vi "MiniWheel Simple Control Code Revised.vi"() -> ()   [LabVIEW 2016]
uses:
  <userlib>/dynamixel/dynamixel.lvlib
panel:
  in  "Baud Rate":i32=1
  in  "Com Port":i32=3
  in  "Goal Omega 2":u16=512 max=1023 step=1
  in  "Goal position 3":u16=512 max=1023 step=1
  in  "Wheel Dynamixel ID":i32=1
  out "Motor Position V. Time":i32(graph)
  in  "Rotator Dynamixel ID":i32=1
  in  "stop":bool
  out "Present Position":u16(slide) max=1023 scale=0.0..1023.0
  # "Instructions:\n1) Enter Initialization Parameters\n2) Enter Goal Omega and Goal Position\n3) Click \"START Motors\" button\n4) Change parameter values as desired during operation"
  # "Motor Feedback"
  # "Initialization"
  # "Parameters"
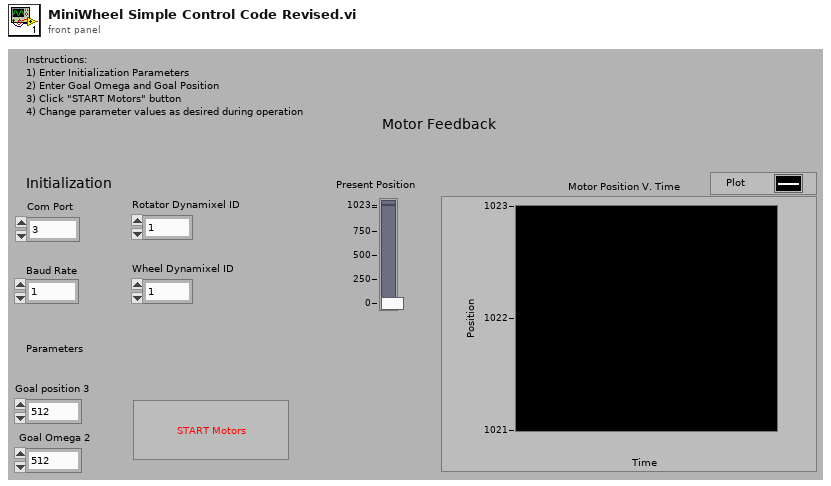
[diagram p1: front panel]
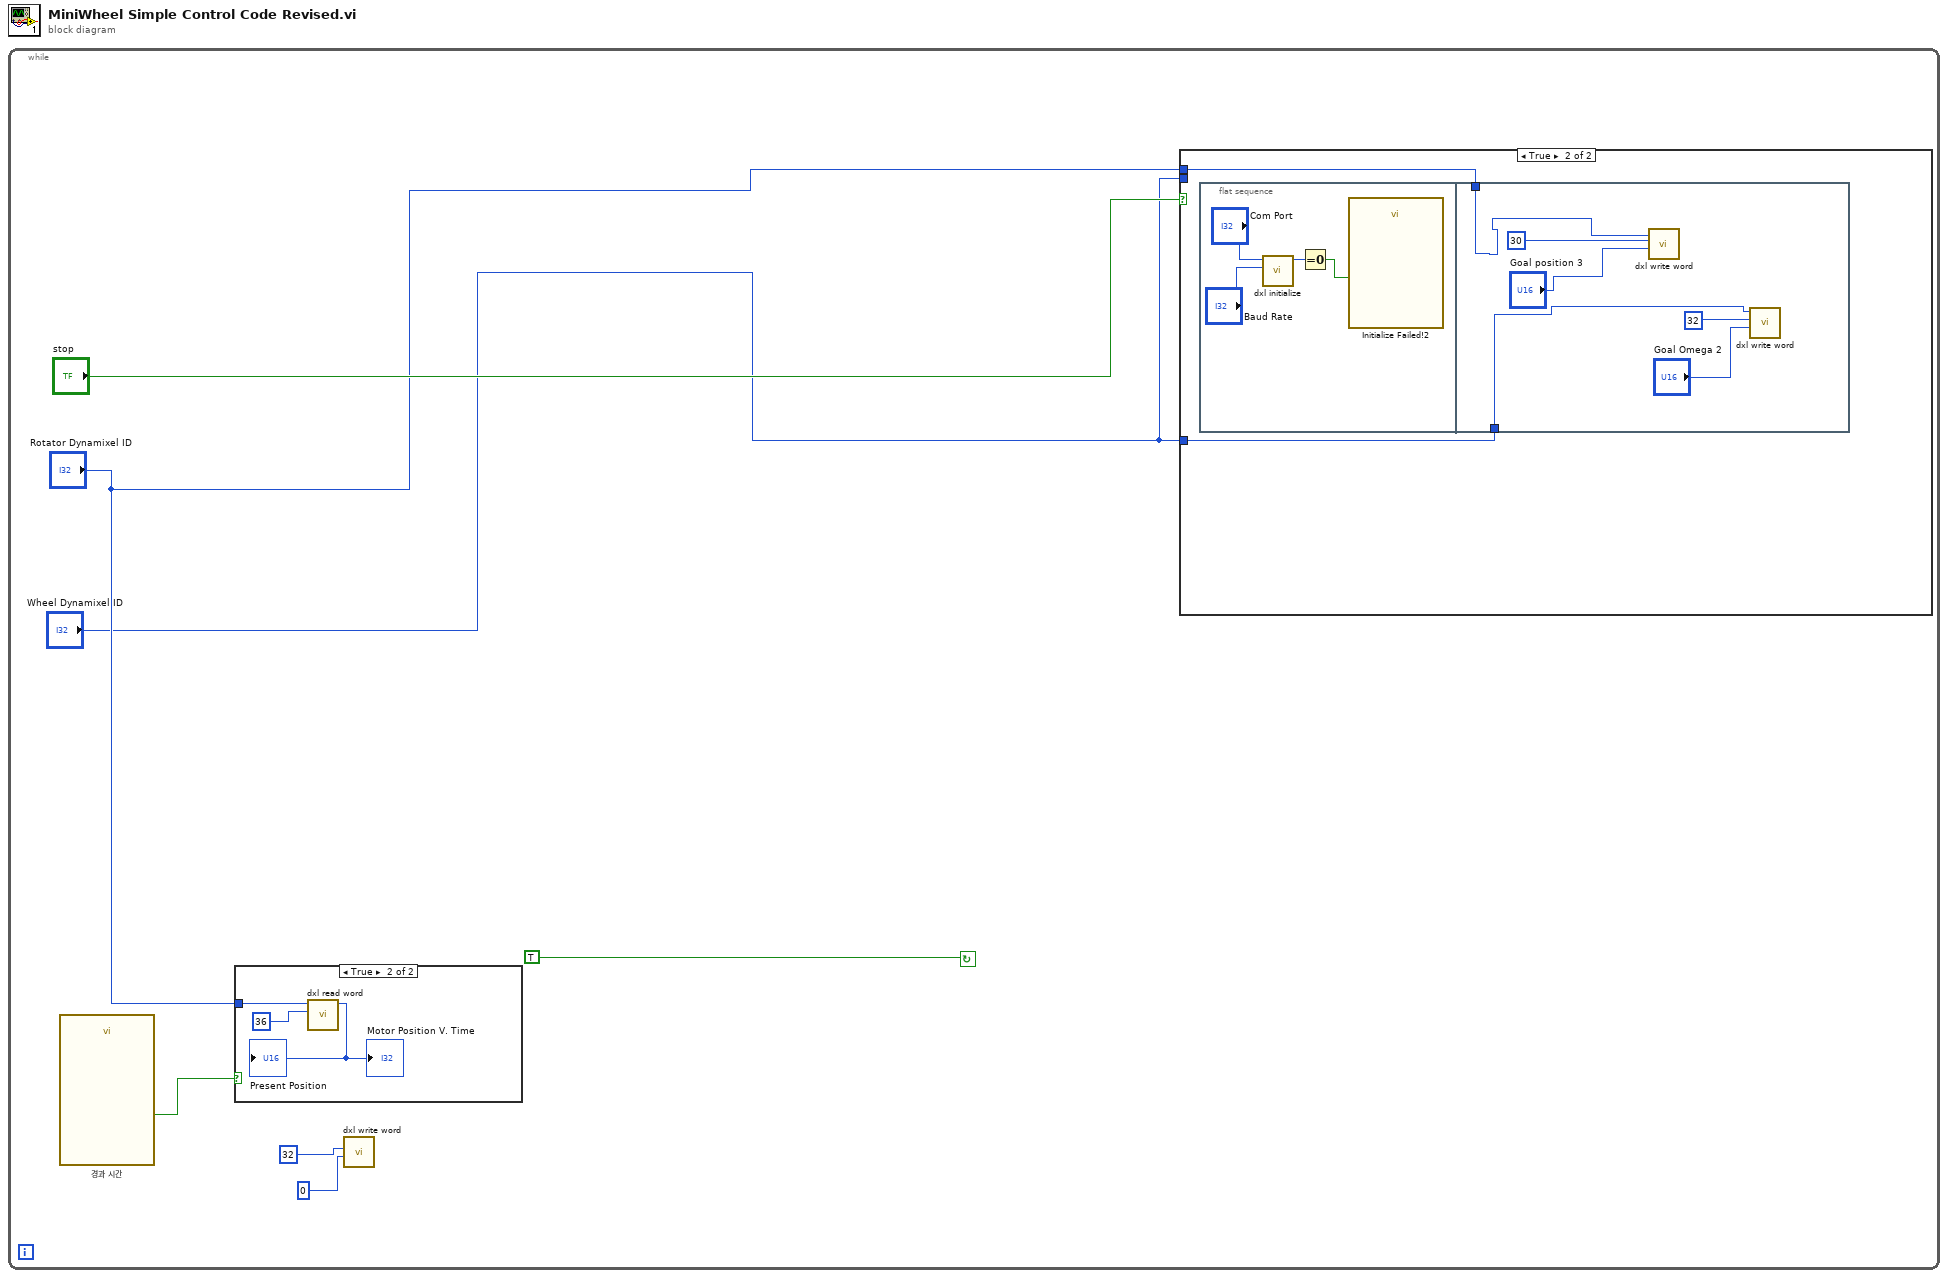
[diagram p0: block diagram]
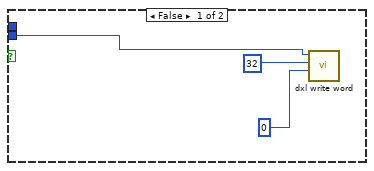
[diagram p2: hidden frame]
diagram:
  n1 = while {
    stop <- TRUE continue-if-true
    n2 = call "경과 시간"() -> ("Time has Elapsed"=w6:bool)  [unwired: 12 in, 7 out]
    n3 = case shown="True" w6 {
      tunnel: "Rotator Dynamixel ID" -> [_ w25]
      frame False {
      }
      frame True {
        n4 = call <userlib>:"dxl read word.vi"("address"=36, "id"=w25) -> ("function return"=→"Present Position" →"Motor Position V. Time":i32)  [unwired: 9 in]
      }
    }
    n5 = call <userlib>:"dxl write word.vi"("value"=0, "address"=32) -> ()  [unwired: 10 in]
    n6 = case shown="True" "stop" {
      tunnel: "Wheel Dynamixel ID" -> [w9 _]
      tunnel: "Rotator Dynamixel ID" -> [_ w12]
      tunnel: "Wheel Dynamixel ID" -> [_ w11]
      frame False {
        n7 = call <userlib>:"dxl write word.vi"("value"=0, "address"=32, "id"=w9) -> ()  [unwired: 9 in]
      }
      frame True {
        n8 = flat-sequence {
          tunnel: w12 -> [w18]
          tunnel: w11 -> [w17]
          frame #0 {
            n9 = call <userlib>:"dxl initialize.vi"("baudnum"="Baud Rate", "devIndex"="Com Port") -> ("function return"=w15:i32)  [unwired: 9 in]
            n10 = Equal To 0?(x=w15) -> (x = 0?=w16:bool)
            n11 = call "Initialize Failed!2"("Enable"=w16) -> ()  [unwired: 9 in, 2 out]
          }
          frame #1 {
            n12 = call <userlib>:"dxl write word.vi"("value"="Goal position 3", "address"=30, "id"=w18) -> ()  [unwired: 9 in]
            n13 = call <userlib>:"dxl write word.vi"("value"="Goal Omega 2", "address"=32, "id"=w17) -> ()  [unwired: 9 in]
          }
        }
      }
    }
  }
